vi "Joystick Test Code.vi"() -> ()   [LabVIEW 2015, in "RDS Libraries.lvlib"]
uses:
  Libraries/Geo/RDS Libraries.lvlib
  <vilib>/Utility/inputDevices.llb/joystickAcquire.vi
panel:
  out "Output":dbl
  in  "stop":bool
  out "output variable":dbl
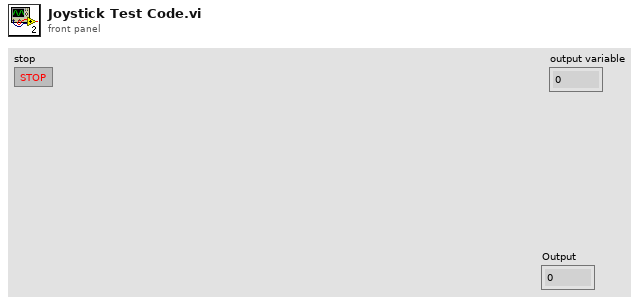
[diagram p1: front panel]
types:
  T1 = cluster{"X axis":i32, "Y axis":i32, "Z axis":i32, "X axis rotation":i32, "Y axis rotation":i32, "Z axis rotation":i32, "U axis":i32, "V axis":i32}
  T2 = cluster{"button 1":bool, "button 2":bool, "button 3":bool, "button 4":bool, "button 5":bool, "button 6":bool, "button 7":bool, "button 8":bool, "button 9":bool, "button 10":bool, "button 11":bool, "button 12":bool, "button 13":bool, "button 14":bool, "button 15":bool, "button 16":bool, "button 17":bool, "button 18":bool, "button 19":bool, "button 20":bool, "button 21":bool, "button 22":bool, "button 23":bool, "button 24":bool, "button 25":bool, "button 26":bool, "button 27":bool, "button 28":bool, "button 29":bool, "button 30":bool, "button 31":bool, "button 32":bool}
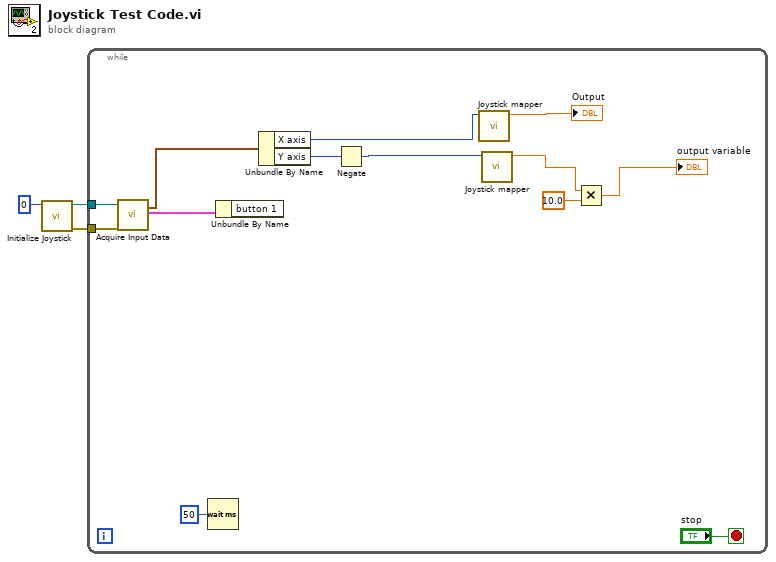
[diagram p0: block diagram]
diagram:
  n1 = call <vilib>:"Initialize Joystick.vi"("device index"=0) -> ("error out"=w1:errorcluster, "device ID"=w2:refnum<k1>)  [unwired: 1 in, 8 out]
  n2 = while {
    tunnel: w2 -> [w16]
    tunnel: w1 -> [w15]
    stop <- "stop" stop-if-true
    n3 = call-poly <vilib>:"Acquire Input Data.vi"("device ID"=w16, "error in (no error)"=w15) -> ("axis info"=w13:T1, "button info"=w4:T2)  [unwired: 16 out]
    n4 = Wait (ms)(milliseconds to wait=u32 50) -> ()  [unwired: 1 out]
    n5 = Unbundle By Name(w4) -> ()  [unwired: 1 out]
    n6 = Unbundle By Name(w13) -> ("X axis"=w9:i32, "Y axis"=w12:i32)
    n7 = Negate(x=w12) -> (-x=w11:i32)
    n8 = call "Joystick mapper.vi"("Input"=w9) -> ("Output"=→"Output":dbl)  [unwired: 10 in]
    n9 = call "Joystick mapper.vi"("Input"=w11) -> ("Output"=w6:dbl)  [unwired: 10 in]
    n10 = Multiply(x=w6, y=10.0) -> (x*y=→"output variable":dbl)
  }
